vi "TWIN_v15_6.vi"() -> ()   [LabVIEW 2017]
uses:
  BERTTA/x64/Debug/BERTTA.dll
panel:
  in  "Log time interval (s)":dbl=20.0 caption="Time Target (s)"
  in  "Add comment":string
  in  "OK Button":bool
  out "Started:":string
  in  "SHUTDOWN":bool
  in  "MASTER CONTROL":bool
  in  "Tab Control":T1(tab)
  out "Output File":path caption="selected path"
  in  "Browse folder":path=path "C:/Users/shresplab/Desktop" caption="start path"
  in  "Read Seq":bool
  in  "Save Seq":bool
  in  "Configuration file":path caption="Filename"
  in  "OK Button 2":bool
  out "Boolean":bool
  in  "User (initials)":string
  in  "Project name":string
  in  "Description":string
  out "Waveform Chart 9":dynamicdata(graph)
  out "Sensor OK 10":bool
  out "Sensor OK 9":bool
  out "Sensor OK 8":bool
  out "Sensor OK 7":bool
  out "Tr 2":dbl format="Tr:              %#_4g"
  out "Tj in 2":dbl format="Tj in:        %#_4g"
  out "Tj out 2":dbl format="Tj out:        %#_4g"
  out "T set 2":dbl format="T set:          %#_4g"
  out "Current step 3":i32 format="Current step:  %.0f"
  out "RPM 6":dbl format="RPM:          %#_g"
  out "Torque 4":dbl format="Torque:      %#_g"
  out "T external 5":dbl format="T (S2):       %#_4g"
  out "PUMP3 2":bool
  out "Led11 17":bool
  out "Target amount 2":dbl
  out "Scale weight 2":dbl
  out "Amount now 3":dbl
  out "Flow rate 2":dbl
  out "Time to target 5":dbl format="%<%H:%M:%S>t"
  out "Current step 2":dbl
  out "Target 2":dbl
  out "Amount now 2":dbl
  out "Led11 12":bool
  out "Target amount":dbl
  out "Scale weight":dbl
  out "Amount now":dbl
  out "Flow rate":dbl
  out "Time to target":dbl format="%<%H:%M:%S>t"
  out "Current step":dbl
  out "Target":dbl
  out "Amount now":dbl
  out "PUMP3":bool
  out "Led11 11":bool
  out "Amount now":dbl
  out "Target":dbl
  out "Current step":dbl
  out "Time to target":dbl format="%<%H:%M:%S>t"
  out "Flow rate":dbl
  out "Amount now":dbl
  out "Scale weight":dbl
  out "Target amount":dbl
  out "PUMP2":bool
  out "Target amount":dbl format="Target amount:        %#_g"
  out "Scale weight":dbl format="Scale weight:     %#_4g"
  out "Amount now":dbl format="Amount now:      %#_4g"
  out "Flow rate":dbl format="Flow rate:                   %#_4g"
  out "Time to target":dbl format="Time to target:     %<%H:%M:%S>t"
  out "Current step":dbl format="Current step:              %#_g"
  out "Target":dbl format="Target:                %#_4g"
  out "Amount now":dbl format="Amount now:    %#_4g"
  out "Led11 10":bool
  out "PUMP1":bool
  out "Sensor OK 6":bool
  out "Sensor OK 5":bool
  out "Sensor OK 4":bool
  out "Sensor OK 3":bool
  out "Tr":dbl format="Tr:              %#_4g"
  out "Tj in":dbl format="Tj in:        %#_4g"
  out "Tj out":dbl format="Tj out:        %#_4g"
  out "T set":dbl format="T set:          %#_4g"
  out "Current step":i32 format="Current step:  %.0f"
  out "RPM":dbl format="RPM:          %#_g"
  out "Torque 2":dbl format="Torque:      %#_g"
  out "T external 3":dbl format="T (S2):       %#_4g"
  out "Waveform Chart 5":dynamicdata(graph)
  out "Waveform Chart 6":dynamicdata(graph)
  out "Waveform Chart 7":dynamicdata(graph)
  in  "OK Button 11":bool=TRUE
  out "Table":string[][](table)=[["14.8.2017 18.06.59", "0,000000", "417,670000", "-0,150000", "1,000000", "22,220000", "23,366837", "23,574959", "23,985852", "23,690000", "240,000000", "4,000000", "0,000000", "397,000000", "-397,000000", "1,000000"], ["14.8.2017 18.07.06", "0,000000", "417,640000", "-0,120000", "1,000000", "22,220000", "23,763115", "23,906257", "23,985694", "23,680000", "240,000000", "4,000000", "0,000000", "397,000000", "-397,000000", "1,000000"], ["14.8.2017 18.07.13", "0,000000", "417,640000", "-0,120000", "1,000000", "22,220000", "23,965922", "24,013440", "23,984906", "23,670000", "240,000000", "4,100000", "3,000000", "397,000000", "-397,000000", "1,000000"], ["14.8.2017 18.07.21", "0,000000", "417,640000", "-0,120000", "1,000000", "22,220000", "23,943860", "23,900110", "23,987113", "23,670000", "240,000000", "4,000000", "0,000000", "397,000000", "-397,000000", "1,000000"], ["14.8.2017 18.07.28", "0,000000", "417,640000", "-0,120000", "1,000000", "22,220000", "23,736328", "23,600018", "23,989004", "23,660000", "240,000000", "4,000000", "0,000000", "397,000000", "-397,000000", "1,000000"], ["14.8.2017 18.07.36", "0,000000", "417,640000", "-0,120000", "1,000000", "22,220000", "23,480910", "23,324538", "23,991053", "23,660000", "240,000000", "4,000000", "0,000000", "397,000000", "-397,000000", "1,000000"], ["14.8.2017 18.07.43", "0,000000", "417,640000", "-0,120000", "2,000000", "22,220000", "23,195579", "23,008270", "23,999093", "23,650000", "240,000000", "4,000000", "0,000000", "397,000000", "-397,000000", "1,000000"], ["14.8.2017 18.07.51", "0,000000", "417,650000", "-417,650000", "1,000000", "22,220000", "22,862541", "22,649021", "24,003979", "23,650000", "240,000000", "4,000000", "0,000000", "397,000000", "-397,000000", "2,000000"], ["14.8.2017 18.07.58", "0,000000", "417,640000", "0,010000", "1,000000", "22,220000", "22,541353", "22,354878", "24,005398", "23,650000", "240,000000", "4,000000", "0,000000", "397,000000", "-397,000000", "1,000000"], ["14.8.2017 18.08.06", "0,000000", "417,640000", "0,010000", "1,000000", "22,220000", "22,347931", "22,253738", "24,007605", "23,640000", "240,000000", "4,100000", "0,000000", "397,000000", "-397,000000", "1,000000"], ["14.8.2017 18.08.13", "0,000000", "417,640000", "0,010000", "1,000000", "22,220000", "22,329030", "22,302102", "24,006028", "23,640000", "240,000000", "4,000000", "0,000000", "395,820000", "-395,820000", "1,000000"], ["14.8.2017 18.08.20", "0,000000", "417,640000", "0,010000", "1,000000", "22,220000", "22,466849", "22,511320", "24,002403", "23,630000", "240,000000", "4,000000", "0,000000", "395,830000", "-0,010000", "1,000000"], ["14.8.2017 18.08.28", "0,000000", "417,640000", "0,010000", "1,000000", "22,220000", "22,707062", "22,835101", "24,000984", "23,620000", "240,000000", "4,000000", "0,000000", "395,830000", "-0,010000", "1,000000"], ["14.8.2017 18.08.35", "0,000000", "417,640000", "0,010000", "1,000000", "22,220000", "23,054104", "23,232979", "24,001299", "23,600000", "240,000000", "4,000000", "0,000000", "395,830000", "-0,010000", "1,000000"], ["14.8.2017 18.08.43", "0,000000", "417,640000", "0,010000", "1,000000", "22,220000", "23,412371", "23,522793", "24,002560", "23,590000", "240,000000", "4,000000", "0,000000", "395,820000", "0,000000", "1,000000"], ["14.8.2017 18.08.51", "0,000000", "417,640000", "0,010000", "1,000000", "22,220000", "23,596247", "23,656125", "24,003821", "23,580000", "240,000000", "4,000000", "0,000000", "395,820000", "0,000000", "1,000000"]]
  out "LED_5 2":bool
  out "LED_4 2":bool
  in  "PAUSE/RUN 11":bool
  in  "TEMP RAMP 2":dbl[][](array[numeric])
  out "LED_3 2":bool
  out "LED_2 2":bool
  out "LED_1 2":bool
  out "LED_MANUAL 2":bool
  in  "Reset 9":bool
  in  "Manual/Ramp 2":bool=TRUE
  in  "Sensor selector 2":bool=TRUE
  in  "Tr/Tj mode selector 2":bool=TRUE
  out "LED STOP 2":bool
  in  "Failsafe 2":dbl=20.0 format="Failsafe temperature:            %#_g"
  out "Current temp 2":dbl format="Current temperature S1:       %#_4g"
  out "Sensor OK 2":bool
  out "T external 4":dbl format="Current temperature S2:       %#_4g"
  in  "OK Button 10":bool
  out "Waveform Chart 2":dynamicdata(graph)
  out "LED_5":bool
  out "LED_4":bool
  in  "PAUSE/RUN 4":bool
  in  "TEMP RAMP":dbl[][](array[numeric])
  out "LED_3":bool
  out "LED_2":bool
  out "LED_1":bool
  out "LED_MANUAL":bool
  in  "Reset 6":bool
  in  "Manual/Ramp":bool=TRUE
  in  "Sensor selector":bool=TRUE
  in  "Tr/Tj mode selector":bool=TRUE
  out "LED STOP":bool
  in  "Failsafe":dbl=20.0 format="Failsafe temperature:            %#_g"
  out "Current temp":dbl format="Current temperature S1:       %#_4g"
  out "Sensor OK":bool
  out "T external 2":dbl format="Current temperature S2:       %#_4g"
  in  "OK Button 3":bool
  out "Waveform Chart":dynamicdata(graph)
  in  "X scales":i64(slide)=50 scale=0.0..100.0
  out "Waveform Chart 19":dynamicdata(graph)
  in  "CLEAR":bool
  in  "ENABLE":bool=TRUE
  out "Led11 16":bool
  out "Led11 15":bool
  in  "PAUSE/RUN 12":bool
  in  "Tube select 4":u32(ring) items=["Big tube", "Double big tube", "Medium tube", "Small tube"]
  in  "Reset 10":bool
  out "Led11 14":bool
  in  "?":bool
  in  "Grams / min 4":dbl
  out "RPM 5":dbl format="%_4f"
  out "Flow rate (g/min) 4":dbl
  out "Scale reading 4":dbl
  out "Step amount now 4":dbl
  out "Total amount now 4":dbl
  out "Elapsed / step 4":dbl format="%<%H:%M:%S>t"
  out "Time to target 4":dbl format="%<%H:%M:%S>t"
  out "Led5 6":bool
  out "Led4 7":bool
  out "Led3 6":bool
  out "Led2 6":bool
  out "Led1 6":bool
  in  "PumpSeq 7":dbl[][](array[numeric])=[[0.0, 0.0, 0.0, 0.0, 0.0, 0.0, 0.0, 0.0, 0.0, 0.0], [0.0, 0.0, 0.0, 0.0, 0.0, 0.0, 0.0, 0.0, 0.0, 0.0], [0.0, 0.0, 0.0, 0.0, 0.0, 0.0, 0.0, 0.0, 0.0, 0.0], [0.0, 0.0, 0.0, 0.0, 0.0, 0.0, 0.0, 0.0, 0.0, 0.0], [0.0, 0.0, 0.0, 0.0, 0.0, 0.0, 0.0, 0.0, 0.0, 0.0], [0.0, 0.0, 0.0, 0.0, 0.0, 0.0, 0.0, 0.0, 0.0, 0.0], [0.0, 0.0, 0.0, 0.0, 0.0, 0.0, 0.0, 0.0, 0.0, 0.0], [0.0, 0.0, 0.0, 0.0, 0.0, 0.0, 0.0, 0.0, 0.0, 0.0], [0.0, 0.0, 0.0, 0.0, 0.0, 0.0, 0.0, 0.0, 0.0, 0.0], [0.0, 0.0, 0.0, 0.0, 0.0, 0.0, 0.0, 0.0, 0.0, 0.0]]
  out "Led11 13":bool
  in  "PAUSE/RUN 9":bool=TRUE
  out "Led11 7":bool
  out "Led11 6":bool
  in  "PAUSE/RUN 3":bool
  in  "Tube select 3":u32(ring) items=["Big tube", "Double big tube", "Medium tube", "Small tube"]
  in  "Reset 8":bool
  out "Led11 9":bool
  in  "?":bool
  in  "Grams / min 3":dbl
  out "RPM 3":dbl format="%_4f"
  out "Flow rate (g/min) 3":dbl
  out "Scale reading 3":dbl
  out "Step amount now 3":dbl
  out "Total amount now 3":dbl
  out "Elapsed / step 3":dbl format="%<%H:%M:%S>t"
  out "Time to target 3":dbl format="%<%H:%M:%S>t"
  out "Led5 5":bool
  out "Led4 5":bool
  out "Led3 5":bool
  out "Led2 5":bool
  out "Led1 5":bool
  in  "PumpSeq 6":dbl[][](array[numeric])=[[0.0, 0.0, 0.0, 0.0, 0.0, 0.0, 0.0, 0.0, 0.0, 0.0], [0.0, 0.0, 0.0, 0.0, 0.0, 0.0, 0.0, 0.0, 0.0, 0.0], [0.0, 0.0, 0.0, 0.0, 0.0, 0.0, 0.0, 0.0, 0.0, 0.0], [0.0, 0.0, 0.0, 0.0, 0.0, 0.0, 0.0, 0.0, 0.0, 0.0], [0.0, 0.0, 0.0, 0.0, 0.0, 0.0, 0.0, 0.0, 0.0, 0.0], [0.0, 0.0, 0.0, 0.0, 0.0, 0.0, 0.0, 0.0, 0.0, 0.0], [0.0, 0.0, 0.0, 0.0, 0.0, 0.0, 0.0, 0.0, 0.0, 0.0], [0.0, 0.0, 0.0, 0.0, 0.0, 0.0, 0.0, 0.0, 0.0, 0.0], [0.0, 0.0, 0.0, 0.0, 0.0, 0.0, 0.0, 0.0, 0.0, 0.0], [0.0, 0.0, 0.0, 0.0, 0.0, 0.0, 0.0, 0.0, 0.0, 0.0]]
  out "Led11 8":bool
  in  "PAUSE/RUN 8":bool=TRUE
  out "Led11 7":bool
  out "Led11 6":bool
  in  "PAUSE/RUN 2":bool
  in  "Tube select 2":u32(ring) items=["Big tube", "Double big tube", "Medium tube", "Small tube"]
  out "Led11 7":bool
  in  "?":bool
  in  "Grams / min 2":dbl
  out "RPM 2":dbl format="%_4f"
  out "Flow rate (g/min) 2":dbl
  out "Scale reading 2":dbl
  out "Step amount now 2":dbl
  out "Total amount now 2":dbl
  out "Elapsed / step 2":dbl format="%<%H:%M:%S>t"
  out "Time to target 2":dbl format="%<%H:%M:%S>t"
  out "Led5 4":bool
  out "Led4 4":bool
  out "Led3 4":bool
  out "Led2 4":bool
  out "Led1 4":bool
  in  "PumpSeq 5":dbl[][](array[numeric])=[[0.0, 0.0, 0.0, 0.0, 0.0, 0.0, 0.0, 0.0, 0.0, 0.0], [0.0, 0.0, 0.0, 0.0, 0.0, 0.0, 0.0, 0.0, 0.0, 0.0], [0.0, 0.0, 0.0, 0.0, 0.0, 0.0, 0.0, 0.0, 0.0, 0.0], [0.0, 0.0, 0.0, 0.0, 0.0, 0.0, 0.0, 0.0, 0.0, 0.0], [0.0, 0.0, 0.0, 0.0, 0.0, 0.0, 0.0, 0.0, 0.0, 0.0], [0.0, 0.0, 0.0, 0.0, 0.0, 0.0, 0.0, 0.0, 0.0, 0.0], [0.0, 0.0, 0.0, 0.0, 0.0, 0.0, 0.0, 0.0, 0.0, 0.0], [0.0, 0.0, 0.0, 0.0, 0.0, 0.0, 0.0, 0.0, 0.0, 0.0], [0.0, 0.0, 0.0, 0.0, 0.0, 0.0, 0.0, 0.0, 0.0, 0.0], [0.0, 0.0, 0.0, 0.0, 0.0, 0.0, 0.0, 0.0, 0.0, 0.0]]
  out "Led11 6":bool
  in  "Reset 7":bool
  in  "PAUSE/RUN 7":bool=TRUE
  out "Led5 7":bool
  out "Led4 6":bool
  in  "PAUSE/RUN":bool
  in  "Tube select":u32(ring) items=["Big tube", "Double big tube", "Medium tube", "Small tube"]
  out "Led11 5":bool
  out "RPM":dbl format="RPM                      %_4f"
  out "Flow rate (g/min)":dbl format="Flow rate               %#_g"
  out "Scale reading":dbl format="Scale reading       %#_g"
  out "Step amount now":dbl format="Step amount       %#_g"
  out "Total amount now":dbl format="Total amount      %#_g"
  out "Elapsed / step":dbl format="Elapsed / step      %<%H:%M:%S>t"
  out "Time to target":dbl format="Time to target     %<%H:%M:%S>t"
  out "Led5 3":bool
  out "Led4 3":bool
  out "Led3 3":bool
  out "Led2 3":bool
  out "Led1 3":bool
  in  "PumpSeq 4":dbl[][](array[numeric])=[[0.0, 0.0, 0.0, 0.0, 0.0, 0.0, 0.0, 0.0, 0.0, 0.0], [0.0, 0.0, 0.0, 0.0, 0.0, 0.0, 0.0, 0.0, 0.0, 0.0], [0.0, 0.0, 0.0, 0.0, 0.0, 0.0, 0.0, 0.0, 0.0, 0.0], [0.0, 0.0, 0.0, 0.0, 0.0, 0.0, 0.0, 0.0, 0.0, 0.0], [0.0, 0.0, 0.0, 0.0, 0.0, 0.0, 0.0, 0.0, 0.0, 0.0], [0.0, 0.0, 0.0, 0.0, 0.0, 0.0, 0.0, 0.0, 0.0, 0.0], [0.0, 0.0, 0.0, 0.0, 0.0, 0.0, 0.0, 0.0, 0.0, 0.0], [0.0, 0.0, 0.0, 0.0, 0.0, 0.0, 0.0, 0.0, 0.0, 0.0], [0.0, 0.0, 0.0, 0.0, 0.0, 0.0, 0.0, 0.0, 0.0, 0.0], [0.0, 0.0, 0.0, 0.0, 0.0, 0.0, 0.0, 0.0, 0.0, 0.0]]
  in  "?":bool
  in  "Grams / min":dbl format="Manual g/min:  %#_g"
  out "Led11 4":bool
  in  "Reset 5":bool
  out "Waveform Chart 18":dynamicdata(graph)
  in  "OK Button 4":bool
  out "Waveform Chart 16":dynamicdata(graph)
  in  "OK Button 5":bool
  out "Waveform Chart 17":dynamicdata(graph)
  in  "OK Button 6":bool
  in  "PAUSE/RUN 5":bool
  in  "?":bool
  in  "Scale port":dbl=5.0
  out "Waveform Chart 15":dynamicdata(graph)
  in  "OK Button 8":bool
  out "RPM 2":dbl
  out "Torque 2":dbl
  out "Waveform Chart 8":dynamicdata(graph)
  in  "OK Button 9":bool
  out "RPM":dbl
  out "Torque":dbl
  out "Waveform Chart 4":dynamicdata(graph)
  in  "OK Button 7":bool
  in  "CDAQ 1 Temp Control 2":tag="EASY9217_2"
  in  "PORT PUMP3 2":i32 format="PUMP 4 PORT:  %.0f"
  in  "SCALE 4":i32 format="SCALE 4 PORT:  %.0f"
  in  "HEIDOLPH 2":i32=3 format="HEIDOLPH 2 PORT:  %.0f"
  in  "LAUDA 2":i32=2 format="LAUDA 2 PORT:  %.0f"
  in  "CDAQ 1 Temp Control":tag="EASY9217_1"
  in  "CDAQ PAM Control":tag="EASY9747"
  in  "PORT PUMP2":i32 format="PUMP 2 PORT:  %.0f"
  in  "PORT PUMP3":i32 format="PUMP 3 PORT:  %.0f"
  in  "PORT PUMP1":i32 format="PUMP 1 PORT:  %.0f"
  in  "Save PortDev":bool
  in  "LAUDA":i32 format="LAUDA 1 PORT:  %.0f"
  in  "HEIDOLPH":i32 format="HEIDOLPH 1 PORT:  %.0f"
  in  "SCALE1":i32 format="SCALE 1 PORT:  %.0f"
  in  "SCALE2":i32 format="SCALE 2 PORT:  %.0f"
  in  "SCALE 3":i32 format="SCALE 3 PORT:  %.0f"
  # "Sensor:"
  # "Control:"
  # "Sensor:"
  # "Control:"
  # "PUMP & SCALE 4"
  # "STEP"
  # "TOTAL"
  # "PUMP & SCALE 3"
  # "STEP"
  # "TOTAL"
  # "PUMP & SCALE 2"
  # "STEP"
  # "TOTAL"
  # "PUMP & SCALE 1"
  # "STEP"
  # "TOTAL"
  # "MANUAL"
  # "RAMP"
  # "Temp Target       Time Target          Wait Time"
  # "STOP"
  # "MANUAL"
  # "RAMP"
  # "Temp Target       Time Target          Wait Time"
  # "STOP"
  # "g              min"
  # "g              min"
  # "g              min"
  # "g              min"
  # "PAM control"
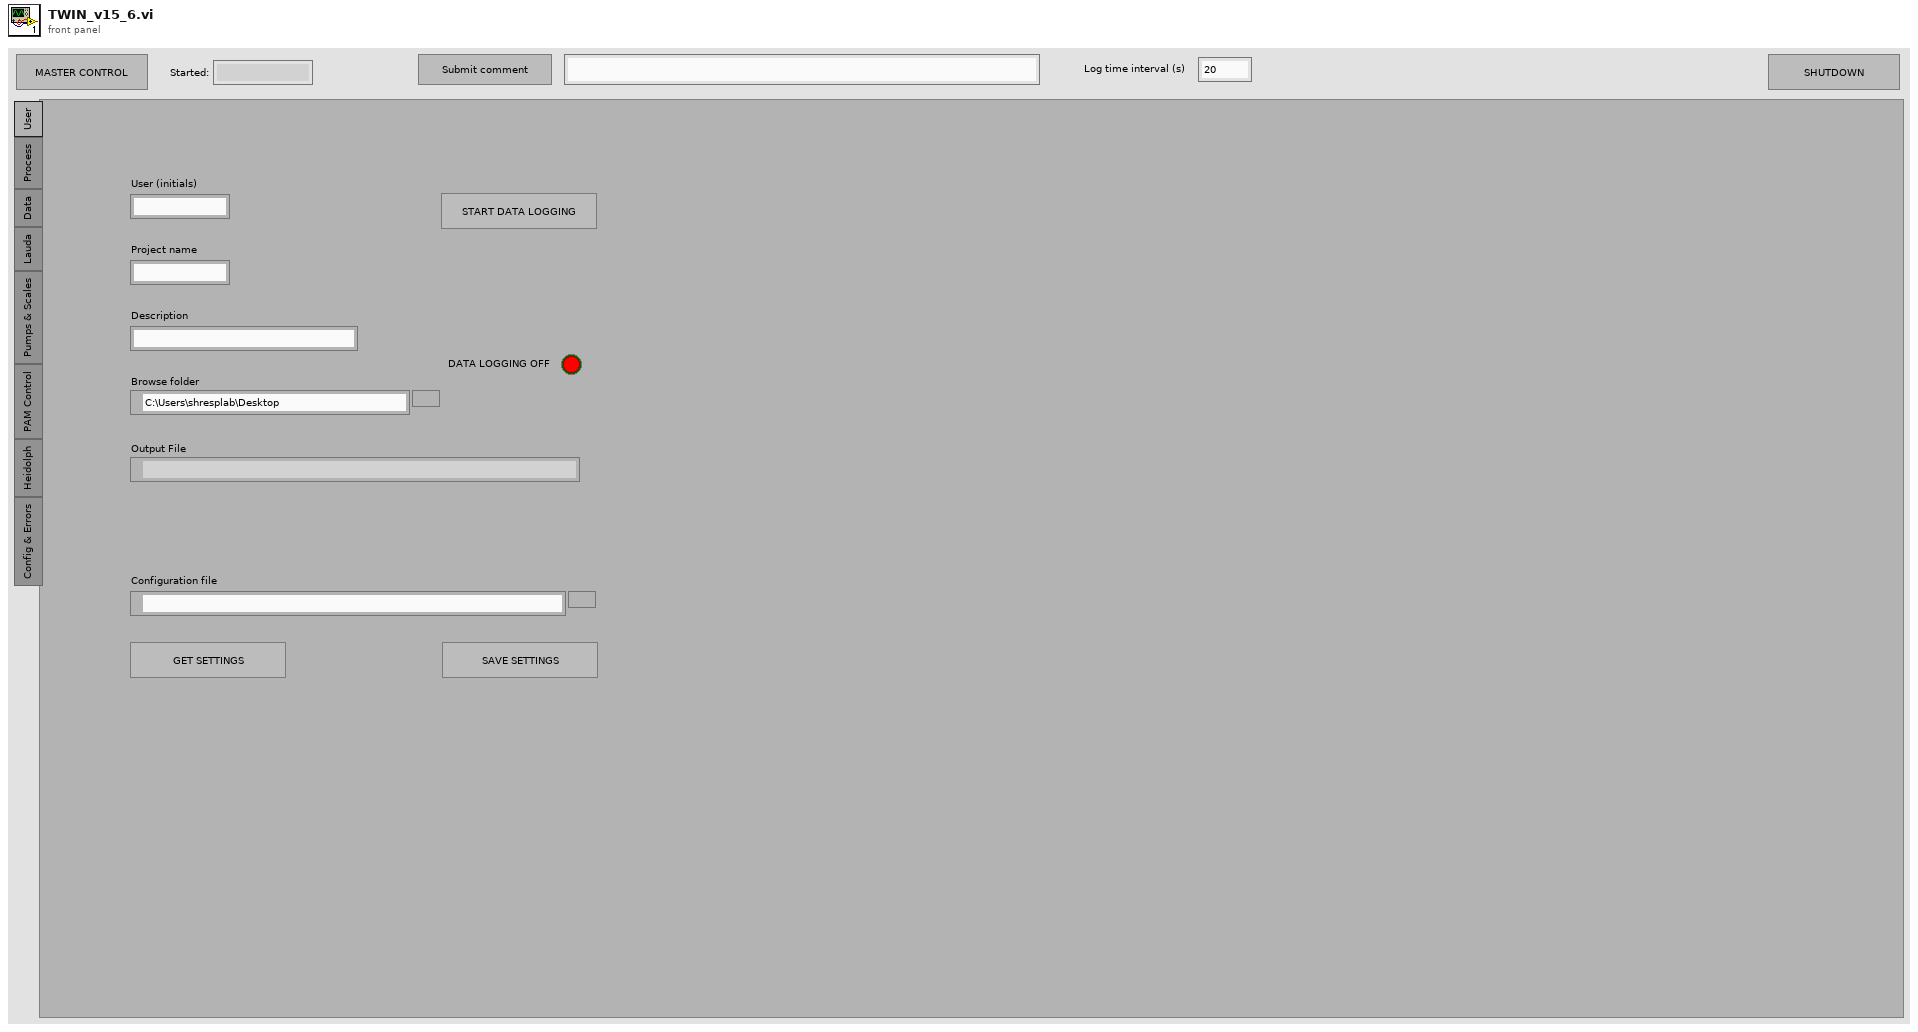
[diagram p1: front panel]
types:
  T1 = enum32{"User", "Process", "Data", "Lauda", "Pumps & Scales", "PAM Control", "Heidolph", "Config & Errors"}
diagram:
  n1 = while {
    i -> [w289]
    stop <- FALSE stop-if-true
    w225 = i64 1000 ("y")
    # "SCALE & PUMP 3"
    n2 = control-ref of="This VI"() -> (w217:refnum<vi>)
    n3 = call "shutdown sequence.vi"("SHUTDOWN"="SHUTDOWN", "VI in"=w217) -> ()  [unwired: 10 in]
    n4 = Not(x="MASTER CONTROL") -> (.not. x?=w324:bool)
    n5 = Boolean To (0,1)(Boolean="PAUSE/RUN 7") -> (0, 1=w22:i16)
    n6 = Boolean To (0,1)(Boolean="PAUSE/RUN 8") -> (0, 1=w21:i16)
    n7 = Boolean To (0,1)(Boolean="PAUSE/RUN 9") -> (0, 1=w20:i16)
    n8 = Boolean To (0,1)(Boolean="ENABLE") -> (0, 1=w19:i16)
    n9 = Multiply(x="X scales", y=w225) -> (x*y=w226:i64)
    n10 = Boolean To (0,1)(Boolean=w324) -> (0, 1=w325:i16)
    n11 = call "RampCTRL_1.vi"("TEMP RAMP"="TEMP RAMP", "Reset 6"="Reset 6") -> ("Array"=w248:dbl[], "Array 2"=w249:dbl[], "Array 3"=w250:dbl[])  [unwired: 7 in]
    n12 = Add(x=w226, y=w225) -> (x+y=w76:i64)
    n13 = for {
      N: w325 -> [_]
      n14 = Get Date/Time String(want seconds? (F)=TRUE) -> (time string=→"Started:":string)  [unwired: 2 in, 1 out]
    }
    n15 = Boolean To (0,1)(Boolean="Sensor selector") -> (0, 1=w243:i16)
    n16 = feedback #1() -> (w224:i64)  [unwired: 1 in]
    n17 = feedback-in #1(w76) -> ()
    n18 = Boolean To (0,1)(Boolean="SHUTDOWN") -> (0, 1=w216:i16)
    n19 = Boolean To (0,1)(Boolean="Reset 6") -> (0, 1=w260:i16)
    n20 = property on="Waveform Chart 2" class="WFChart (strict)"() -> ("History Data"=w78:dynamicdata[])  [unwired: 2 in, 2 out]
    n21 = Not Equal?(x=w224, y=w76) -> (x != y?=w223:bool)
    n22 = property on="Waveform Chart" class="WFChart (strict)"() -> ("History Data"=w228:dynamicdata[])  [unwired: 2 in, 2 out]
    n23 = call "ReadMoxa12.vi"("PORT 1"="LAUDA", "PORT 2"="LAUDA 2", "PORT 3"="HEIDOLPH", "PORT 4"="HEIDOLPH 2", "PORT 5"="SCALE1", "PORT 6"="SCALE2", "PORT 7"="SCALE 3", "PORT 8"="SCALE 4", "enable1"=w22, "enable2"=w21, "enable3"=w20, "enable4"=w19) -> ("params"=w62:dbl[])  [unwired: 7 in]
    n24 = Boolean To (0,1)(Boolean=w223) -> (0, 1=w221:i16)
    n25 = Array Size(array=w228) -> (size(s)=w222:i32)
    n26 = Array Size(array=w78) -> (size(s)=w77:i32)
    n27 = Boolean To (0,1)(Boolean="Tr/Tj mode selector") -> (0, 1=w244:i16)
    n28 = call "SensorMode1.vi"("Numeric"=w243, "Numeric 2"=w244) -> ("Sensor OK 4"=→"Sensor OK 4":bool, "Sensor OK 5"=→"Sensor OK 5":bool, "Sensor OK 6"=→"Sensor OK 6":bool, "Sensor OK 3"=→"Sensor OK 3":bool)  [unwired: 6 in]
    n29 = for {
      N: w221 -> [_]
      tunnel: w222 -> [w351]
      tunnel: w76 -> [w350]
      tunnel: w77 -> [w347]
      tunnel: w76 -> [w346]
      n30 = Add(x=w347, y=w346) -> (x+y=w348:i64)
      n31 = Add(x=w351, y=w350) -> (x+y=w349:i64)
      n32 = property on="Waveform Chart" class="WFChart (strict)"("XScale.Maximum"=w349) -> ()  [unwired: 2 in, 2 out]
      n33 = property on="Waveform Chart 2" class="WFChart (strict)"("XScale.Maximum"=w348) -> ()  [unwired: 2 in, 2 out]
    }
    n34 = Boolean To (0,1)(Boolean="Manual/Ramp") -> (0, 1=w258:i16)
    n35 = And(x="MASTER CONTROL", y="PAUSE/RUN 4") -> (x .and. y?=w257:bool)
    n36 = Build Array("LAUDA", "LAUDA 2", "HEIDOLPH", "HEIDOLPH 2", "SCALE1", "SCALE2", "SCALE 3", "SCALE 4", "PORT PUMP1", "PORT PUMP2", "PORT PUMP3", "PORT PUMP3 2") -> (w232:i32[])
    n37 = Boolean To (0,1)(Boolean=w257) -> (0, 1=w256:i16)
    n38 = call "LaudaDAQ.vi"("device name"="CDAQ 1 Temp Control") -> (1:"Tj out"=→"Tj out":dbl, "data"=w318:dynamicdata, "Sensor OK"=→"Sensor OK":bool, 4:"Tj out"=→"Tj in":dbl, "T external 2"=w218:dbl)  [unwired: 5 in, 1 out]
    "T external 2" <- w218
    "T external 3" <- w218
    n39 = Boolean To (0,1)(Boolean="Save PortDev") -> (0, 1=w292:i16)
    n40 = for {
      N: w292 -> [_]
      tunnel: w232 -> [w405]
      tunnel: "Save PortDev" -> [w406]
      n41 = call "Convert to Dynamic Data"("Array"=w405) -> ("Dynamic Data Type"=w404:dynamicdata)  [unwired: 3 in]
      n42 = call "Write To Measurement File3"("Signals"=w404, "Reset"=w406) -> ()  [unwired: 15 in, 3 out]
    }
    n43 = Boolean To (0,1)(Boolean="OK Button 9") -> (0, 1=w80:i16)
    n44 = for {
      N: w80 -> [_]
      n45 = property on="Waveform Chart 8" class="WFChart (strict)"("History Data"=dynamicdata[] []) -> ()  [unwired: 2 in, 2 out]
    }
    n46 = Less?(x=w289, y=1.0) -> (x < y?=w287:bool)
    n47 = call "HEI_Data.vi"("params"=w62) -> ("Waveform Chart 8"=→"Waveform Chart 8":dynamicdata, "RPM"=w16:dbl, "Dynamic Data"=w57:dynamicdata, "RPM 2"=w10:dbl, "RPM 6"=→"RPM 6":dbl, "Torque 4"=→"Torque 4":dbl, "Torque 2"=→"Torque 2":dbl, "Waveform Chart 4"=→"Waveform Chart 4":dynamicdata, "Torque 3"=→"Torque 2":dbl, "Torque"=→"Torque":dbl, "RPM 4"=→"RPM 2":dbl, "Waveform Chart 6"=→"Waveform Chart 6":dynamicdata)  [unwired: 7 in]
    "RPM" <- w16
    "RPM" <- w10
    n48 = Equal?(x=w16, y=0.0) -> (x = y?=w15:bool)
    n49 = Boolean To (0,1)(Boolean=w15) -> (0, 1=w14:i16)
    n50 = call "Fail_Clock_1.vi"("fail"=w14) -> ("Trigger"=w18:dbl)  [unwired: 10 in]
    n51 = call "Ramp_Lauda_v3.vi"("manual"=w258, "Tr_Tj"=w244, "shutdown"=w216, "S1_S2"=w243, "Tr"=w62, "T_fail"="Failsafe", "fail"=w18, "enable"=w256, "time_set"=w249, "reset"=w260, "time_wait"=w248, "T_S2"=w218, "port"="LAUDA", "T_sp"=w250) -> ("LED_1"=→"LED_1":bool, "LED_manual"=→"LED_MANUAL":bool, "LED_2"=→"LED_2":bool, "step"=w235:dbl, "LED_stop"=→"LED STOP":bool, "LED_3"=→"LED_3":bool, "LED 4"=→"LED_4":bool, "LED 5"=→"LED_5":bool, "setpoint"=w24:dbl, "Tr_out"=w255:dbl, "T int"=w254:dbl)  [unwired: 1 in, 2 out]
    "Tr" <- w255
    "T set" <- w24
    "Current temp" <- w255
    n52 = Add(x=w235, y=1.0) -> (x+y=→"Current step":dbl)
    n53 = Equal?(x=w10, y=0.0) -> (x = y?=w12:bool)
    n54 = Boolean To (0,1)(Boolean=w12) -> (0, 1=w11:i16)
    n55 = Merge Signals(w24, w255, w254, w318) -> (w37:dynamicdata)
    "Waveform Chart" <- w37
    "Waveform Chart 5" <- w37
    n56 = call "Fail_Clock_2.vi"("fail"=w11) -> ("Trigger"=w9:dbl)  [unwired: 10 in]
    n57 = Boolean To (0,1)(Boolean=w287) -> (0, 1=w288:i16)
    n58 = for {
      N: w288 -> [_]
      tunnel: w287 -> [w399]
      n59 = while {
        tunnel: [w402] -> w398
        tunnel: w399 -> [w400]
        stop <- w403 stop-if-true
        n60 = call "Read From Measurement File2"("Enable"=TRUE, "Reset"=w400) -> ("Signals"=w402:dynamicdata, "EOF?"=w403:bool)  [unwired: 4 in, 4 out]
      }
      n61 = call "Convert from Dynamic Data2"("Dynamic Data Type"=w398) -> ("Array"=w374:dbl[])  [unwired: 3 in]
      n62 = Index Array(array=w374, index=0) -> (element=w391:dbl)
      n63 = Index Array(array=w374, index=1) -> (element=w380:dbl)
      n64 = Index Array(array=w374, index=2) -> (element=w390:dbl)
      n65 = Index Array(array=w374, index=3) -> (element=w378:dbl)
      n66 = Index Array(array=w374, index=4) -> (element=w389:dbl)
      n67 = Index Array(array=w374, index=5) -> (element=w388:dbl)
      n68 = Index Array(array=w374, index=6) -> (element=w387:dbl)
      n69 = Index Array(array=w374, index=7) -> (element=w376:dbl)
      n70 = Index Array(array=w374, index=8) -> (element=w382:dbl)
      n71 = Index Array(array=w374, index=9) -> (element=w384:dbl)
      n72 = Index Array(array=w374, index=10) -> (element=w383:dbl)
      n73 = Index Array(array=w374, index=11) -> (element=w373:dbl)
      n74 = property on="LAUDA" class="DigNum (strict)"("Val(Sgnl)"=w391) -> ()  [unwired: 2 in, 2 out]
      n75 = property on="LAUDA 2" class="DigNum (strict)"("Val(Sgnl)"=w380) -> ()  [unwired: 2 in, 2 out]
      n76 = property on="HEIDOLPH" class="DigNum (strict)"("Val(Sgnl)"=w390) -> ()  [unwired: 2 in, 2 out]
      n77 = property on="HEIDOLPH 2" class="DigNum (strict)"("Val(Sgnl)"=w378) -> ()  [unwired: 2 in, 2 out]
      n78 = property on="SCALE1" class="DigNum (strict)"("Val(Sgnl)"=w389) -> ()  [unwired: 2 in, 2 out]
      n79 = property on="SCALE2" class="DigNum (strict)"("Val(Sgnl)"=w388) -> ()  [unwired: 2 in, 2 out]
      n80 = property on="SCALE 3" class="DigNum (strict)"("Val(Sgnl)"=w387) -> ()  [unwired: 2 in, 2 out]
      n81 = property on="SCALE 4" class="DigNum (strict)"("Val(Sgnl)"=w376) -> ()  [unwired: 2 in, 2 out]
      n82 = property on="PORT PUMP1" class="DigNum (strict)"("Val(Sgnl)"=w382) -> ()  [unwired: 2 in, 2 out]
      n83 = property on="PORT PUMP2" class="DigNum (strict)"("Val(Sgnl)"=w384) -> ()  [unwired: 2 in, 2 out]
      n84 = property on="PORT PUMP3" class="DigNum (strict)"("Val(Sgnl)"=w383) -> ()  [unwired: 2 in, 2 out]
      n85 = property on="PORT PUMP3 2" class="DigNum (strict)"("Val(Sgnl)"=w373) -> ()  [unwired: 2 in, 2 out]
    }
    n86 = Boolean To (0,1)(Boolean="OK Button 3") -> (0, 1=w299:i16)
    n87 = Boolean To (0,1)(Boolean="Reset 9") -> (0, 1=w123:i16)
    n88 = for {
      N: w299 -> [_]
      n89 = property on="Waveform Chart" class="WFChart (strict)"("History Data"=dynamicdata[] []) -> ()  [unwired: 2 in, 2 out]
    }
    n90 = call "RampCTRL_2.vi"("TEMP RAMP in"="TEMP RAMP 2", "Reset 9"="Reset 9") -> ("Array"=w115:dbl[], "Array 2"=w116:dbl[], "Array 3"=w117:dbl[])  [unwired: 7 in]
    n91 = And(x="MASTER CONTROL", y="PAUSE/RUN 11") -> (x .and. y?=w130:bool)
    n92 = Boolean To (0,1)(Boolean="Manual/Ramp 2") -> (0, 1=w126:i16)
    n93 = Boolean To (0,1)(Boolean="Tr/Tj mode selector 2") -> (0, 1=w75:i16)
    n94 = Boolean To (0,1)(Boolean="Sensor selector 2") -> (0, 1=w74:i16)
    n95 = call "SensorMode2.vi"("Numeric"=w74, "Numeric 2"=w75) -> ("Sensor OK 8"=→"Sensor OK 8":bool, "Sensor OK 10"=→"Sensor OK 10":bool, "Sensor OK 9"=→"Sensor OK 9":bool, "Sensor OK 7"=→"Sensor OK 7":bool)  [unwired: 6 in]
    n96 = Boolean To (0,1)(Boolean=w130) -> (0, 1=w129:i16)
    n97 = call "LaudaDAQ2.vi"("device name"="CDAQ 1 Temp Control 2") -> (1:"Tj out"=→"Tj out 2":dbl, "data"=w54:dynamicdata, "Sensor OK"=→"Sensor OK 2":bool, 4:"Tj out"=→"Tj in 2":dbl, "T external 2"=→"T external 4" →"T external 5":dbl)  [unwired: 5 in, 1 out]
    n98 = call "Ramp_Lauda_v3_2.vi"("manual"=w126, "Tr_Tj"=w75, "S1_S2"=w74, "Tr"=w62, "T_fail"="Failsafe 2", "fail"=w9, "enable"=w129, "time_set"=w116, "reset"=w123, "time_wait"=w115, "port"="LAUDA 2", "T_sp"=w117) -> ("LED_1"=→"LED_1 2":bool, "LED_manual"=→"LED_MANUAL 2":bool, "LED_2"=→"LED_2 2":bool, "step"=w121:dbl, "LED_stop"=→"LED STOP 2":bool, "LED_3"=→"LED_3 2":bool, "LED 4"=→"LED_4 2":bool, "LED 5"=→"LED_5 2":bool, "setpoint"=w23:dbl, "Tr_out"=w114:dbl, "T int"=w113:dbl)  [unwired: 3 in, 2 out]
    "Current temp 2" <- w114
    "T set 2" <- w23
    "Tr 2" <- w114
    n99 = Boolean To (0,1)(Boolean="OK Button 4") -> (0, 1=w297:i16)
    n100 = Add(x=w121, y=1.0) -> (x+y=→"Current step 3":dbl)
    n101 = for {
      N: w297 -> [_]
      n102 = property on="Waveform Chart 18" class="WFChart (strict)"("History Data"=dynamicdata[] []) -> ()  [unwired: 2 in, 2 out]
    }
    n103 = Merge Signals(w23, w114, w113, w54) -> (w36:dynamicdata)
    "Waveform Chart 2" <- w36
    "Waveform Chart 9" <- w36
    n104 = Boolean To (0,1)(Boolean="OK Button 5") -> (0, 1=w241:i16)
    n105 = for {
      N: w241 -> [_]
      n106 = property on="Waveform Chart 16" class="WFChart (strict)"("History Data"=dynamicdata[] []) -> ()  [unwired: 2 in, 2 out]
    }
    n107 = call "IsmaCTRL.vi"("FR_manual"="Grams / min", "tube selector"="Tube select", "Manual"="?", "Reset"="Reset 5", "Pause"="PAUSE/RUN", "Setpoint_W   /   Setpoint_T"="PumpSeq 4", "Enable"="MASTER CONTROL", "Scale"=w62) -> ("Boolean 9"=→"Led11 5" →"Led11 10":bool, "Boolean"=→"Led1 3":bool, "Boolean 2"=→"Led2 3":bool, "Total target"=→"Target":dbl, "Boolean 3"=→"Led3 3":bool, "Boolean 4"=→"Led4 3":bool, "lastAmount"=→"Step amount now":dbl, "step"=→"Current step":dbl, "Boolean 5"=→"Led5 3":bool, "Boolean 6"=→"Led4 6":bool, "Boolean 7"=→"Led5 7":bool, "FR"=w199:dbl, "RPM"=w60:dbl, "Weight"=w195:dbl, "elapsed"=→"Elapsed / step":dbl, "time_to_target"=→"Time to target" →"Time to target":dbl, "pumpCTRL"=w211:dbl, "Target_step"=→"Target amount":dbl, "Boolean 8"=w203:bool)  [unwired: 1 out]
    "Flow rate" <- w199
    "Scale weight" <- w195
    "Led11 4" <- w203
    "Scale reading" <- w195
    "Flow rate (g/min)" <- w199
    "RPM" <- w60
    n108 = Boolean To (0,1)(Boolean="OK Button 6") -> (0, 1=w239:i16)
    n109 = for {
      N: w239 -> [_]
      n110 = property on="Waveform Chart 17" class="WFChart (strict)"("History Data"=dynamicdata[] []) -> ()  [unwired: 2 in, 2 out]
    }
    n111 = Multiply(x=w195, y=-1.0 ("x")) -> (x*y=→"Amount now" →"Amount now" →"Total amount now":dbl)
    n112 = And(x="PAUSE/RUN", y=w203) -> (x .and. y?=w277:bool)
    n113 = feedback #2() -> (w278:bool)  [unwired: 1 in]
    n114 = feedback-in #2(w277) -> ()
    n115 = Greater?(x=w211, y=70.0) -> (0:→"PUMP1":bool)
    n116 = Not Equal?(x=w278, y=w277) -> (x != y?=w276:bool)
    n117 = Boolean To (0,1)(Boolean=w276) -> (0, 1=w275:i16)
    n118 = for {
      N: w275 -> [_]
      n119 = property on="PAUSE/RUN" class="Bool (strict)"("Val(Sgnl)"=FALSE ("Value (Signaling)")) -> ()  [unwired: 2 in, 2 out]
    }
    n120 = Merge Signals(w195, w199) -> (w242:dynamicdata)
    "Waveform Chart 18" <- w242
    n121 = Boolean To (0,1)(Boolean="OK Button 7") -> (0, 1=w295:i16)
    n122 = for {
      N: w295 -> [_]
      n123 = property on="Waveform Chart 4" class="WFChart (strict)"("History Data"=dynamicdata[] []) -> ()  [unwired: 2 in, 2 out]
    }
    n124 = call "IsmaCTRL_2.vi"("FR_manual"="Grams / min 2", "tube selector"="Tube select 2", "Manual"="?", "Reset"="Reset 7", "Pause"="PAUSE/RUN 2", "Setpoint_W   /   Setpoint_T"="PumpSeq 5", "Enable"="MASTER CONTROL", "Scale"=w62) -> ("Boolean 9"=→"Led11 7" →"Led11 11":bool, "Boolean"=→"Led1 4":bool, "Boolean 2"=→"Led2 4":bool, "Total target"=→"Target":dbl, "Boolean 3"=→"Led3 4":bool, "Boolean 4"=→"Led4 4":bool, "lastAmount"=→"Amount now" →"Step amount now 2":dbl, "step"=→"Current step":dbl, "Boolean 5"=→"Led5 4":bool, "Boolean 6"=→"Led11 6":bool, "Boolean 7"=→"Led11 7":bool, "FR"=w182:dbl, "RPM"=w59:dbl, "Weight"=w183:dbl, "elapsed"=→"Elapsed / step 2":dbl, "time_to_target"=→"Time to target" →"Time to target 2":dbl, "pumpCTRL"=w176:dbl, "Target_step"=→"Target amount":dbl, "Boolean 8"=w166:bool)  [unwired: 1 out]
    "Scale weight" <- w183
    "Flow rate" <- w182
    "Led11 6" <- w166
    "Scale reading 2" <- w183
    "Flow rate (g/min) 2" <- w182
    "RPM 2" <- w59
    n125 = Boolean To (0,1)(Boolean="OK Button 8") -> (0, 1=w284:i16)
    n126 = for {
      N: w284 -> [_]
      n127 = property on="Waveform Chart 15" class="WFChart (strict)"("History Data"=dynamicdata[] []) -> ()  [unwired: 2 in, 2 out]
    }
    n128 = Merge Signals(w183, w182) -> (w272:dynamicdata)
    "Waveform Chart 16" <- w272
    n129 = Multiply(x=w183, y=-1.0) -> (x*y=→"Amount now" →"Total amount now 2":dbl)
    n130 = And(x="PAUSE/RUN 2", y=w166) -> (x .and. y?=w270:bool)
    n131 = Greater?(x=w176, y=70.0) -> (0:→"PUMP2":bool)
    n132 = feedback #3() -> (w271:bool)  [unwired: 1 in]
    n133 = feedback-in #3(w270) -> ()
    n134 = Not Equal?(x=w271, y=w270) -> (x != y?=w269:bool)
    n135 = Boolean To (0,1)(Boolean=w269) -> (0, 1=w268:i16)
    n136 = for {
      N: w268 -> [_]
      n137 = property on="PAUSE/RUN 2" class="Bool (strict)"("Val(Sgnl)"=FALSE ("Value (Signaling)")) -> ()  [unwired: 2 in, 2 out]
    }
    n138 = Boolean To (0,1)(Boolean="CLEAR") -> (0, 1=w83:i16)
    n139 = for {
      N: w83 -> [_]
      n140 = property on="Waveform Chart 19" class="WFChart (strict)"("History Data"=dynamicdata[] []) -> ()  [unwired: 2 in, 2 out]
    }
    n141 = call "IsmaCTRL_3.vi"("FR_manual"="Grams / min 3", "tube selector"="Tube select 3", "Manual"="?", "Reset"="Reset 8", "Pause"="PAUSE/RUN 3", "Setpoint_W   /   Setpoint_T"="PumpSeq 6", "Enable"="MASTER CONTROL", "Scale"=w62) -> ("Boolean 9"=→"Led11 9" →"Led11 12":bool, "Boolean"=→"Led1 5":bool, "Boolean 2"=→"Led2 5":bool, "Total target"=→"Target":dbl, "Boolean 3"=→"Led3 5":bool, "Boolean 4"=→"Led4 5":bool, "lastAmount"=→"Amount now" →"Step amount now 3":dbl, "step"=→"Current step":dbl, "Boolean 5"=→"Led5 5":bool, "Boolean 6"=→"Led11 6":bool, "Boolean 7"=→"Led11 7":bool, "FR"=w152:dbl, "RPM"=w58:dbl, "Weight"=w151:dbl, "elapsed"=→"Elapsed / step 3":dbl, "time_to_target"=→"Time to target" →"Time to target 3":dbl, "pumpCTRL"=w157:dbl, "Target_step"=→"Target amount":dbl, "Boolean 8"=w142:bool)  [unwired: 1 out]
    "Scale weight" <- w151
    "Flow rate" <- w152
    "Led11 8" <- w142
    "Scale reading 3" <- w151
    "Flow rate (g/min) 3" <- w152
    "RPM 3" <- w58
    n142 = Multiply(x=w151, y=-1.0) -> (x*y=→"Amount now" →"Total amount now 3":dbl)
    n143 = Merge Signals(w195, w183, w151) -> (→"Waveform Chart 7":dynamicdata)
    n144 = Greater?(x=w157, y=70.0) -> (0:→"PUMP3":bool)
    n145 = And(x="MASTER CONTROL", y=w142) -> (x .and. y?=w263:bool)
    n146 = Merge Signals(w151, w152) -> (w265:dynamicdata)
    "Waveform Chart 17" <- w265
    n147 = feedback #4() -> (w264:bool)  [unwired: 1 in]
    n148 = feedback-in #4(w263) -> ()
    n149 = Not Equal?(x=w264, y=w263) -> (x != y?=w262:bool)
    n150 = Boolean To (0,1)(Boolean=w262) -> (0, 1=w261:i16)
    n151 = for {
      N: w261 -> [_]
      n152 = property on="PAUSE/RUN 3" class="Bool (strict)"("Val(Sgnl)"=FALSE ("Value (Signaling)")) -> ()  [unwired: 2 in, 2 out]
    }
    n153 = call "Convert to Dynamic Data6"("2D Array"="PumpSeq 7") -> ("Dynamic Data Type"=w26:dynamicdata)  [unwired: 3 in]
    n154 = call "Convert to Dynamic Data4"("2D Array"="PumpSeq 6") -> ("Dynamic Data Type"=w305:dynamicdata)  [unwired: 3 in]
    n155 = call "Convert to Dynamic Data3"("2D Array"="PumpSeq 5") -> ("Dynamic Data Type"=w306:dynamicdata)  [unwired: 3 in]
    n156 = call "Convert to Dynamic Data2"("2D Array"="PumpSeq 4") -> ("Dynamic Data Type"=w308:dynamicdata)  [unwired: 3 in]
    n157 = Merge Signals(w26, w305, w306, w308) -> (w307:dynamicdata)
    n158 = call "IsmaCTRL_4.vi"("FR_manual"="Grams / min 4", "tube selector"="Tube select 4", "Manual"="?", "Reset"="Reset 10", "Pause"="PAUSE/RUN 12", "Setpoint_W   /   Setpoint_T"="PumpSeq 7", "Enable"="MASTER CONTROL") -> ("Boolean 9"=→"Led11 14" →"Led11 17":bool, "Boolean"=→"Led1 6":bool, "Boolean 2"=→"Led2 6":bool, "Total target"=→"Target 2":dbl, "Boolean 3"=→"Led3 6":bool, "Boolean 4"=→"Led4 7":bool, "lastAmount"=→"Step amount now 4" →"Amount now 3":dbl, "step"=→"Current step 2":dbl, "Boolean 5"=→"Led5 6":bool, "Boolean 6"=→"Led11 15":bool, "Boolean 7"=→"Led11 16":bool, "FR"=w48:dbl, "RPM"=w56:dbl, "Weight"=w84:dbl, "elapsed"=→"Elapsed / step 4":dbl, "time_to_target"=→"Time to target 4" →"Time to target 5":dbl, "pumpCTRL"=w92:dbl, "Target_step"=→"Target amount 2":dbl, "Boolean 8"=w101:bool)  [unwired: 1 in, 1 out]
    "Led11 13" <- w101
    "Scale reading 4" <- w84
    "Flow rate (g/min) 4" <- w48
    "RPM 5" <- w56
    "Flow rate 2" <- w48
    "Scale weight 2" <- w84
    n159 = call "WriteMoxa12.vi"("PORT LAUDA 1"="LAUDA", "DATA LAUDA 1"=w24, "enable2"=w21, "DATA LAUDA 2"=w23, "DATA ISMA 1"=w60, "PORT LAUDA 2"="LAUDA 2", "DATA ISMA 2"=w59, "enable1"=w22, "enable4"=w19, "PORT ISMA 1"="PORT PUMP1", "DATA ISMA 3"=w58, "PORT ISMA 2"="PORT PUMP2", "PORT ISMA 3"="PORT PUMP3", "PORT ISMA 4"="PORT PUMP3 2", "enable3"=w20, "DATA ISMA 4"=w56) -> ()
    n160 = Boolean To (0,1)(Boolean="Save Seq") -> (0, 1=w304:i16)
    n161 = for {
      N: w304 -> [_]
      tunnel: w307 -> [w441]
      tunnel: "Configuration file" -> [w442]
      tunnel: "Save Seq" -> [w440]
      n162 = call "Write To Measurement File2"("Signals"=w441, "Reset"=w440, "Filename"=w442) -> ()  [unwired: 14 in, 3 out]
    }
    n163 = Multiply(x=w84, y=-1.0) -> (x*y=w85:dbl)
    "Total amount now 4" <- w85
    "Amount now 2" <- w85
    n164 = Greater?(x=w92, y=70.0) -> (0:→"PUMP3 2":bool)
    n165 = And(x="MASTER CONTROL", y=w101) -> (x .and. y?=w104:bool)
    n166 = feedback #5() -> (w105:bool)  [unwired: 1 in]
    n167 = feedback-in #5(w104) -> ()
    n168 = Merge Signals(w85, w48) -> (w38:dynamicdata)
    "Waveform Chart 19" <- w38
    n169 = Not Equal?(x=w105, y=w104) -> (x != y?=w103:bool)
    n170 = Boolean To (0,1)(Boolean=w103) -> (0, 1=w102:i16)
    n171 = for {
      N: w102 -> [_]
      n172 = property on="PAUSE/RUN 12" class="Bool (strict)"("Val(Sgnl)"=FALSE ("Value (Signaling)")) -> ()  [unwired: 2 in, 2 out]
    }
    n173 = Boolean To (0,1)(Boolean="Read Seq") -> (0, 1=w303:i16)
    n174 = for {
      N: w303 -> [_]
      tunnel: "Configuration file" -> [w425]
      tunnel: "Read Seq" -> [w424]
      n175 = while {
        tunnel: [w439] -> w435
        tunnel: w425 -> [w438]
        tunnel: w424 -> [w436]
        stop <- w437 stop-if-true
        n176 = call "Read From Measurement File"("Filename"=w438, "Reset"=w436) -> ("Signals"=w439:dynamicdata, "EOF?"=w437:bool)  [unwired: 4 in, 4 out]
      }
      n177 = call "Convert from Dynamic Data"("Dynamic Data Type"=w435) -> ("Array"=w428:dbl[][])  [unwired: 3 in]
      n178 = Array Subset(array=w428, index (row)=20 ("index"), length (row)=10 ("length")) -> (w421:dbl[][])  [unwired: 2 in]
      n179 = Array Subset(array=w428, index (row)=10 ("index"), length (row)=10 ("length")) -> (w422:dbl[][])  [unwired: 2 in]
      n180 = Array Subset(array=w428, index (row)=0 ("index"), length (row)=10 ("length")) -> (w420:dbl[][])  [unwired: 2 in]
      n181 = Array Subset(array=w428, index (row)=30 ("index"), length (row)=8 ("length")) -> (w423:dbl[][])  [unwired: 2 in]
      n182 = property on="PumpSeq 6" class="Arr (strict)"("Val(Sgnl)"=w422) -> ()  [unwired: 2 in, 2 out]
      n183 = property on="PumpSeq 7" class="Arr (strict)"("Val(Sgnl)"=w420) -> ()  [unwired: 2 in, 2 out]
      n184 = property on="PumpSeq 4" class="Arr (strict)"("Val(Sgnl)"=w423) -> ()  [unwired: 2 in, 2 out]
      n185 = property on="PumpSeq 5" class="Arr (strict)"("Val(Sgnl)"=w421) -> ()  [unwired: 2 in, 2 out]
    }
    n186 = Merge Signals(w242, w272, w265, w38) -> (w319:dynamicdata)
    n187 = Merge Signals(w37, w36, w319, w57) -> (w286:dynamicdata)
    n188 = Boolean To (0,1)(Boolean="PAUSE/RUN 5") -> (0, 1=w246:i16)
    n189 = for {
      N: w246 -> [_]
      tunnel: "MASTER CONTROL" -> [w355]
      tunnel: "PAUSE/RUN 5" -> [w354]
      n190 = And(x=w354, y="?") -> (x .and. y?=w363:bool)
      n191 = dll-call lib="C:/Users/shresplab/OneDrive - Kemira Oyj/Documents/GitHub/Bertta/BERTTA/x64/Debug/BERTTA.dll" fn="mettler"("port"="Scale port", "msg"=1) -> ("return type"=w357:dbl)  [unwired: 5 in, 2 out]
      n192 = And(x=w355, y=w363) -> (x .and. y?=w360:bool)
      n193 = Initialize Array(FALSE, 1 ("dimension size")) -> (w362:bool[])
      n194 = Replace Array Subset(array=w362, new element=w360, index=0) -> (w359:bool[])
      n195 = call "Convert to Dynamic Data5"("Double"=w357) -> ("Dynamic Data Type"=→"Waveform Chart 15":dynamicdata)  [unwired: 3 in]
      n196 = call "DAQ Assistant"("data"=w359, "device name"="CDAQ PAM Control") -> ()  [unwired: 16 in, 2 out]
    }
    n197 = call "filenameparser_09.vi"("Description"="Description", "start path"="Browse folder", "Project name"="Project name", "User (initials)"="User (initials)", "OK Button in"="OK Button 2") -> ("appended path 2"=w293:path, "appended path"=w321:path)  [unwired: 4 in, 1 out]
    "Output File" <- w293
    n198 = feedback #6() -> (w2:i32)  [unwired: 1 in]
    n199 = Equal?(x=1.0, y=w2) -> (x = y?=w4:bool)
    n200 = Boolean To (0,1)(Boolean="OK Button") -> (0, 1=w320:i16)
    n201 = call "Elapsed Time"("Time Target (s)"="Log time interval (s)", "Reset"=w4) -> ("Time has Elapsed"=w6:bool)  [unwired: 10 in, 7 out]
    n202 = for {
      N: w320 -> [_]
      tunnel: w321 -> [w412]
      w416 = " " ("string")
      n203 = property on="Add comment" class="Str"("Val(Sgnl)"="" ("Value (Signaling)")) -> ()  [unwired: 2 in, 2 out]
      n204 = Get Date/Time String(want seconds? (F)=TRUE) -> (date string=w419:string, time string=w417:string)  [unwired: 2 in]
      n205 = Concatenate Strings(w419, w416, w417, w416, "Add comment") -> (w415:string)
      n206 = feedback #7() -> (w414:string[])  [unwired: 1 in]
      n207 = Build Array (concatenate)(w414, w415) -> (w413:string[])
      n208 = feedback-in #7(w413) -> ()
      n209 = Write to Text File(file (use dialog)=w412, text=w413) -> ()  [unwired: 2 in, 3 out]
    }
    n210 = Boolean To (0,1)(Boolean=w6) -> (0, 1=w7:i16)
    n211 = for {
      N: w7 -> [_]
      tunnel: "OK Button 2" -> [w336]
      tunnel: w293 -> [w335]
      tunnel: w286 -> [w333]
      tunnel: [w330] -> w3
      i -> [w330]
      n212 = call "Header Names TWIN.vi"("Dynamic Data"=w333) -> ("Signals Out"=w334:dynamicdata)  [unwired: 10 in]
      n213 = call "Write To Measurement File"("Signals"=w334, "Enable"=w336, "Filename"=w335) -> ()  [unwired: 14 in, 3 out]
      n214 = Boolean To (0,1)(Boolean="OK Button 11") -> (0, 1=w331:i16)
      n215 = for {
        N: w331 -> [_]
        tunnel: w333 -> [w337]
        n216 = call "Build Table"("Include time data"=TRUE, "Signals"=w337) -> ("Table"=w341:string[][])  [unwired: 3 in, 6 out]
        n217 = Delete From Array(array=w341, length=23, index (col)=0 ("index (row)")) -> (array with subset deleted=→"Table":string[][])  [unwired: 1 in, 1 out]
      }
    }
    n218 = feedback-in #6(w3) -> ()
    "Boolean" <- "OK Button 2"
  }
